vi "Write Data to a File.vi"() -> ()   [LabVIEW 2017]
uses:
  UI Error Handlers/support/Logging/Logging.lvlib
panel:
  in  "Boolean":bool
  in  "# of Random Numbers to Write to File":i32
  # "Overview: This example shows two possible methods for writing data to a file to save/log/view later.\nRequirements: LabVIEW 2013 (or compatible)\nInstructions:\n1. Set File location and name of file on the VI's front panel by clicking on the folder icon.\n2. Run VI\n3. Open desired file"
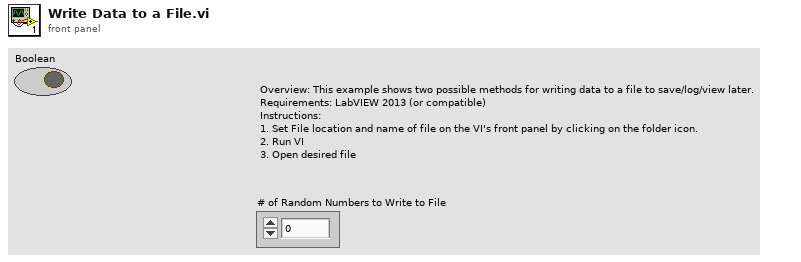
[diagram p1: front panel]
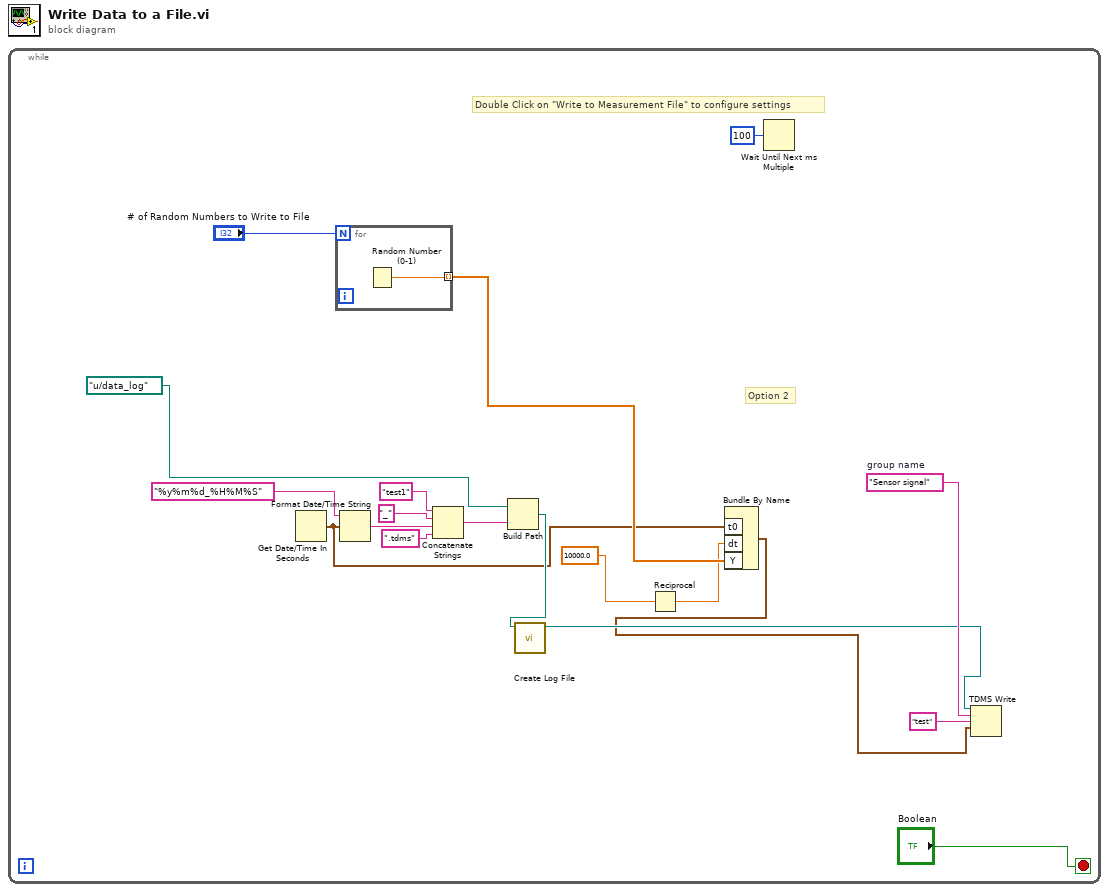
[diagram p0: block diagram]
diagram:
  n1 = while {
    stop <- "Boolean" stop-if-true
    w7 = "Sensor signal"  # group name
    # "Option 2"
    # "Double Click on \"Write to Measurement File\" to configure settings"
    n2 = Get Date/Time In Seconds() -> (seconds since 1Jan1904=w3:timestamp)
    n3 = for {
      N: "# of Random Numbers to Write to File" -> [_]
      tunnel: [w20] -> w10 mode=indexing
      n4 = Random Number (0-1)() -> (number: 0 to 1=w20:dbl)
    }
    n5 = Format Date/Time String(time format string (%c)="%y%m%d_%H%M%S", seconds (now)=w3) -> (date/time string=w17:string)  [unwired: 1 out]
    n6 = Concatenate Strings("test1" ("string"), "_" ("string"), w17, ".tdms" ("string")) -> (w13:string)
    n7 = Build Path(base path=path "u:/data_log" ("AVI Path"), name or relative path=w13) -> (appended path=w11:path)
    n8 = call "Create Log File.vi"("Acceleration Exceeded Log Folder"=w11) -> ("Log File out"=w6:refnum<k34>)  [unwired: 9 in, 1 out]
    n9 = Reciprocal(x=10000.0 ("dt")) -> (1/x=w8:dbl)
    n10 = Bundle By Name("t0"=w3, "dt"=w8, "Y"=w10) -> (w5:waveform(dbl))  [unwired: 1 in]
    n11 = Wait Until Next ms Multiple(millisecond multiple=u32 100) -> ()  [unwired: 1 out]
    n12 = TDMS Write(0:w6, 5:w7, 7:"test" ("channel name(s) in (Untitled)"), 9:w5) -> ()  [unwired: 2 in, 4 out]
  }
